vi "Cambiar Tamaño y tipo de Fuente.vi"   [LabVIEW 2020]
uses:
  <vilib>/Utility/traverseref.llb/TRef TravTarget.ctl
  <vilib>/Utility/miscctls.llb/LVTextColorsTypeDef.ctl
  <vilib>/Utility/traverseref.llb/VI Scripting - Traverse.lvlib
types:
  T1 = typedef "TRef TravTarget.ctl" = enum16{"FP", "BD", "Other"}
  T2 = typedef "LVTextColorsTypeDef.ctl" = cluster{"Text Color":u32, "Background Color":u32}
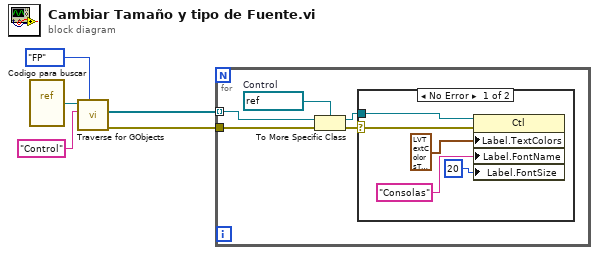
[diagram p0: block diagram]
diagram:
  n1 = vi-ref "Codigo para buscar.vi"() -> (w4:refnum<vi>)
  n2 = call <vilib>:"Traverse for GObjects.vi"("Traverse Target"=TRef_TravTarget."FP", "Class Name"="Control", "VI Refnum"=w4) -> ("error out"=w5:errorcluster, "References"=w1:refnum<vi>[])  [unwired: 5 in, 2 out]
  n3 = for {
    tunnel: w1 -> [w8] mode=indexing
    tunnel: w5 -> [w10]
    w7 = refnum<vi> refnum  # Control
    n4 = To More Specific Class(target class=w7, reference=w8, error in=w10) -> (specific class reference=w6:refnum<vi>, error out=w9:errorcluster)
    n5 = case shown="No Error" w9 {
      selector: w9 -> [w15 _]
      tunnel: w6 -> [w14 _]
      frame No Error {
        n6 = property class="Ctl"(reference=w14, error in=w15, "Label.TextColors"=T2 {"Text Color"=16711680, "Background Color"=16777216} ("Label.Text Colors"), "Label.FontName"="Consolas" ("Label.Font:Name"), "Label.FontSize"=u32 20 ("Label.Font:Size")) -> ()  [unwired: 2 out]
      }
      frame Error {
      }
    }
  }
